vi "Cursor Plane XZ Visible Read.vi"(4 "error in (no error)":errorcluster, 6 "Container State":T3, 7 "Display State In":T1) -> (0 "error out":errorcluster, 2 "Value":bool, 3 "Display State Out":T1)   [LabVIEW 2020, in "3D Bar.xctl"]
uses:
  <vilib>/Math Plots/3D Math Plots/3D Bar/3D Bar XCtrl/3D Bar.xctl
  <vilib>/_xctls/Container State.ctl
  <vilib>/Math Plots/3D Math Plots/3D Bar/3D Bar XCtrl/State.ctl
  <vilib>/Math Plots/3D Math Plots/3D Bar/3D Bar/3D Bar.lvclass
  e:/builds/penguin/labview/branches/2020/dev/dist/vi.lib/Math Plots/3D Math Plots/3D Plot/3D Plot/3D Plot.lvclass
  <vilib>/Math Plots/3D Math Plots/3D Plot/Action String/3DMathPlot Ctrl Act Queue.ctl
  <vilib>/Math Plots/3D Math Plots/3D Plot/Action String/3DMathPlot Ctrl Act Cluster.ctl
  <vilib>/Math Plots/3D Math Plots/3D Plot/Action String/3DMathPlot State Class.ctl
  <vilib>/Math Plots/3D Math Plots/3D Plot/3D Plot/3D Plot.lvclass
  <vilib>/_xctls/XControlSupport.lvlib
panel:
  # "Replace the Value Indicator below with an Indicator of desired type.\nDo not remove this Indicator or the others from the connector pane. \nDo not change the connector pane pattern.\nThe Value Indicator should always be the second terminal from top on the output side in the connector pane."
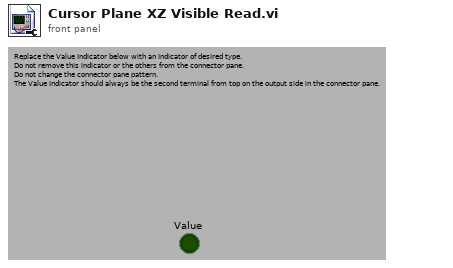
[diagram p1: front panel]
types:
  T1 = typedef "3D Bar.xctl/State.ctl" = cluster{"3D Bar.lvclass":refnum<class "3D Bar.lvclass">, "Control Ref Queue":T2, "Plot Width":u32, "Main Frame Color":u32, "Ramp Palette Color":u32, "Projection Palette Color":u32}
  T2 = typedef "3DMathPlot Ctrl Act Queue.ctl" = refnum<queue>
  T3 = typedef "XControlSupport.lvlib/Container State.ctl" = cluster{"Indicator?":bool, "Run Mode?":bool, " Refnum":refnum<vi>}
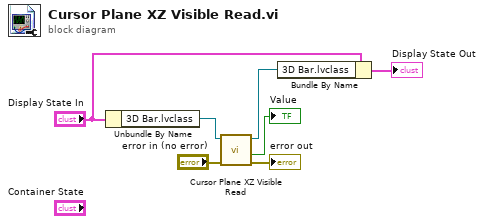
[diagram p0: block diagram]
diagram:
  n1 = Unbundle By Name("Display State In") -> ("3D Bar.lvclass"=w7:refnum<class "3D Bar.lvclass">)
  n2 = call <vilib>:"Cursor Plane XZ Visible Read.vi"("error in (no error)"="error in (no error)", "3D Plot.lvclass in"=w7) -> ("error out"=→"error out":errorcluster, "Plane XZ"=→"Value":bool, "3D Plot.lvclass out"=w3:refnum<class "3D Bar.lvclass">)  [unwired: 7 out]
  n3 = Bundle By Name(cluster="Display State In", "3D Bar.lvclass"=w3) -> (→"Display State Out":T1)
